vi "Timing of Reference Scans.vi"() -> (1 "#image_lines_# = ROUNDUP( ((2ms – tref)/time_image_line)) +1":i32, 2 "Tref(usec)":dbl, 3 "time_image_line (usec)":dbl)   [LabVIEW 2020]
uses:
  Global Variables/General Globals.vi
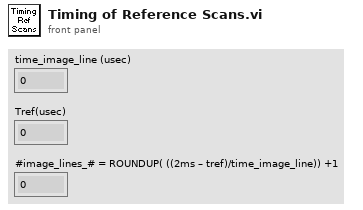
[diagram p1: front panel]
types:
  T1 = typedef "Ref DAQ Param.ctl" = cluster{"Full Frame Size":u16, "Ref Field of View":sgl, "Ref Zoom":i8, "Ref_dwellTime":sgl, "Ref X-pixels-per-line(Npxr)":i16, "Ref Y-lines-per-image(Npyr)":i16, "Ref Z-lines-per-image":i16, "Ignore Z lines":i16, "Ref Scan Cycles":i32, "Ref threshold XY":u16, "Ref threshold Z":u16, "Ref average XY":u16, "Ref Average  Z":u16, "Proportional_scale":fxp<+,16,2>, "Integral_scale":fxp<+/-,16,12>, "Proportional_scale Z":fxp<+,16,2>, "Integral_scale Z":fxp<+/-,16,12>, "Diff_threshold":fxp<+,16,2>, "Diff_threshold _z":fxp<+,16,2>, "Sliding Average":bool, "Ref count reset enabled":bool}
  T2 = typedef "AOL_Globals.ctl" = cluster{"Imaging Protocol":T3, "Number of POI":u16, "Number of Miniscans":u16, "Number of Trials":u16, "Number of Cycles ":u64, "# Averaged Frames":u16, "Laser power (%)":u8, "Pockels (V)":dbl, "Acquisition Length (sec)":dbl, "Fill time (us)":dbl, "POI Dwell time (us)":dbl, "Miniscan Dwell time per pixel (us)":dbl, "PMT 1":dbl, "PMT 2":dbl, "Back Apperture (mA)":dbl, "Frame Size":T4, "Center Frequency":dbl, "Field of View (norm)":dbl, "DwellTime (us)":dbl, "Wavelength (nm)":dbl, "Zoom":dbl, "AOL Z":dbl, "AOL Mode":T5, "GridXY":dbl, "GridZ":dbl, "TriggerPeriod (sec)":dbl, "Number of Pixels in Miniscan":u16, "Experiment folder path":path, "X centre":dbl, "Y centre":dbl, "Angle (degrees)":dbl, "Plane Mode":T6, "Threshold":u16[], "Regenerate Chirps":bool, "Rectangle ROI length (pixels)":u16, "Rectangle ROI height (pixels)":u16, "AOD fill":u16, "StartupDelay":i32, "Samples Wait after Trigger":u16, "Slip Cycle":u32, "Add Cycle":bool, "Functional Mode":T7, "Z Start":dbl, "Z Stop":dbl, "# Planes":i32, "Total Pixels":i32, "Variable Miniscan Pixels":u16[], "Use Variable Length":bool, "Use Variable Resolution":bool, "Laser power (%) at Z Start":u8, "Laser power (%) at Z Stop":u8, "Ref Z Step":i8, "Ref Dwell Time (us)":dbl, "Field of View (um)":dbl}
  T3 = typedef "Imaging Protocols enum.ctl" = enum16{"AOL Z-Stack", "Motor Z Stack", "Functional Acquisition", "Single Plane Acquisition", "Volume Acquisition", "Live Imaging", "Live Plane Imaging", "Live Volume Imaging"}
  T4 = typedef "Frame Size.ctl" = u16
  T5 = typedef "AOL modes.ctl" = enum16{"Raster", "Structural", "Pointing", "Mini Scan", "Alignment"}
  T6 = typedef "Plane Mode.ctl" = u16
  T7 = typedef "Functional Mode.ctl" = enum16{"Point", "Line", "Patch", "Plane", "Volume"}
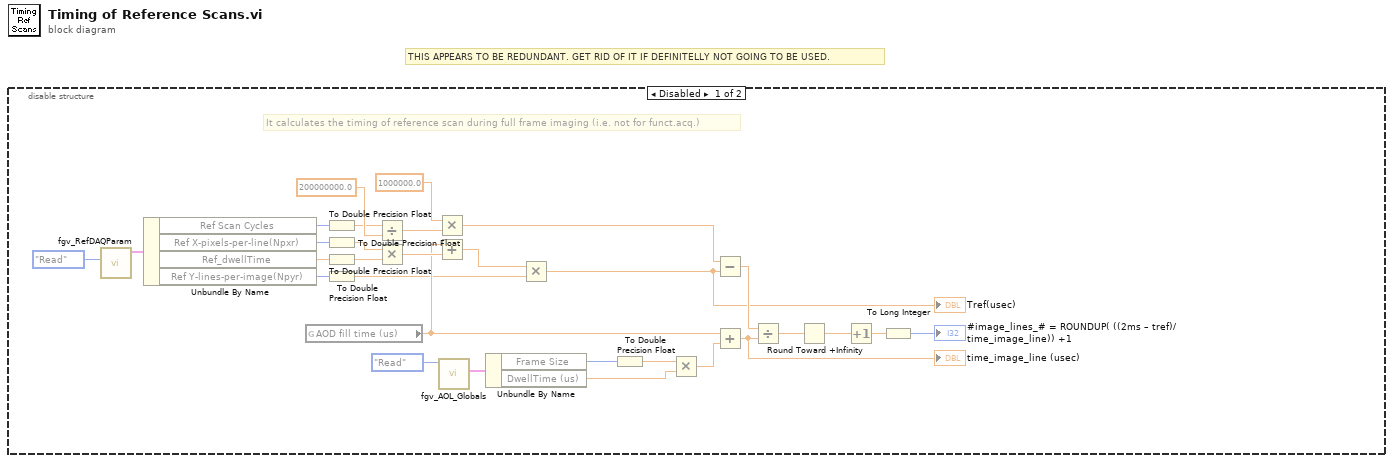
[diagram p0: block diagram]
diagram:
  # "THIS APPEARS TO BE REDUNDANT. GET RID OF IT IF DEFINITELLY NOT GOING TO BE USED."
  n1 = disable-structure shown="Disabled" {
    frame Disabled {
      # "It calculates the timing of reference scan during full frame imaging (i.e. not for funct.acq.)"
      n2 = call "fgv_RefDAQParam.vi"("Function"=enum16{"Initialize", "Write", "Read"}."Read" ("Status")) -> ("RefDAQParam"=w20:T1)  [unwired: 9 in, 1 out]
      n3 = Unbundle By Name(w20) -> ("Ref Scan Cycles"=w13:i32, "Ref X-pixels-per-line(Npxr)"=w19:i16, "Ref_dwellTime"=w18:sgl, "Ref Y-lines-per-image(Npyr)"=w17:i16)
      n4 = global read "General Globals.vi" "AOD fill time (us)"() -> (w22:dbl)
      n5 = To Double Precision Float(number=w13) -> (double precision float=w11:dbl)
      n6 = To Double Precision Float(number=w19) -> (double precision float=w15:dbl)
      n7 = To Double Precision Float(number=w18) -> (double precision float=w14:dbl)
      n8 = To Double Precision Float(number=w17) -> (double precision float=w16:dbl)
      n9 = Divide(x=w11, y=200000000.0) -> (x/y=w10:dbl)
      n10 = Multiply(x=w15, y=w14) -> (x*y=w30:dbl)
      n11 = Multiply(x=1000000.0, y=w10) -> (x*y=w9:dbl)
      n12 = Add(x=w22, y=w30) -> (x+y=w29:dbl)
      n13 = call "fgv_AOL_Globals.vi"("Function"=enum16{"Intialize", "Write", "Read", "Clear"}."Read") -> ("AOL_Globals"=w6:T2)  [unwired: 9 in, 1 out]
      n14 = Unbundle By Name(w6) -> ("Frame Size"=w5:T4, "DwellTime (us)"=w3:dbl)
      n15 = Multiply(x=w29, y=w16) -> (x*y=w1:dbl)
      "Tref(usec)" <- w1
      n16 = To Double Precision Float(number=w5) -> (double precision float=w4:dbl)
      n17 = Multiply(x=w4, y=w3) -> (x*y=w28:dbl)
      n18 = Subtract(x=w9, y=w1) -> (x-y=w27:dbl)
      n19 = Add(x=w22, y=w28) -> (x+y=w23:dbl)
      "time_image_line (usec)" <- w23
      n20 = Divide(x=w27, y=w23) -> (x/y=w26:dbl)
      n21 = Round Toward +Infinity(x=w26) -> (ceil(x): smallest int >= x=w25:dbl)
      n22 = Increment(x=w25) -> (x+1=w24:dbl)
      n23 = To Long Integer(number=w24) -> (32bit integer=→"#image_lines_# = ROUNDUP( ((2ms – tref)/time_image_line)) +1":i32)
    }
    frame Enabled {
    }
  }
